vi "菜单-执行.vi"(8 "error in (no error)":errorcluster caption="错误输入（无错误）", 11 "程序响应 输入":refnum<class "程序响应.lvclass">) -> (0 "error out":errorcluster caption="错误输出", 3 "程序响应 输出":refnum<class "程序响应.lvclass">)   [LabVIEW 2020, in "程序响应.lvlib" / "程序响应.lvclass"]
uses:
  D:/SuperPython-master/ScintillaNET.dll
  ScintillaNET.dll
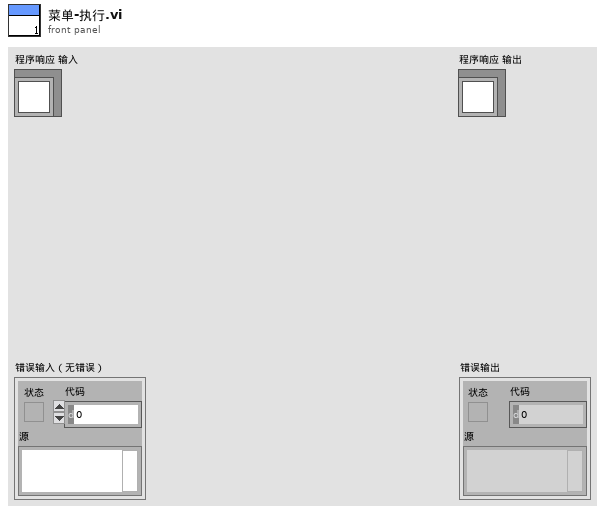
[diagram p1: front panel]
types:
  T1 = enum16{"open", "replace", "create", "open or create", "replace or create", "replace or create with confirmation"}
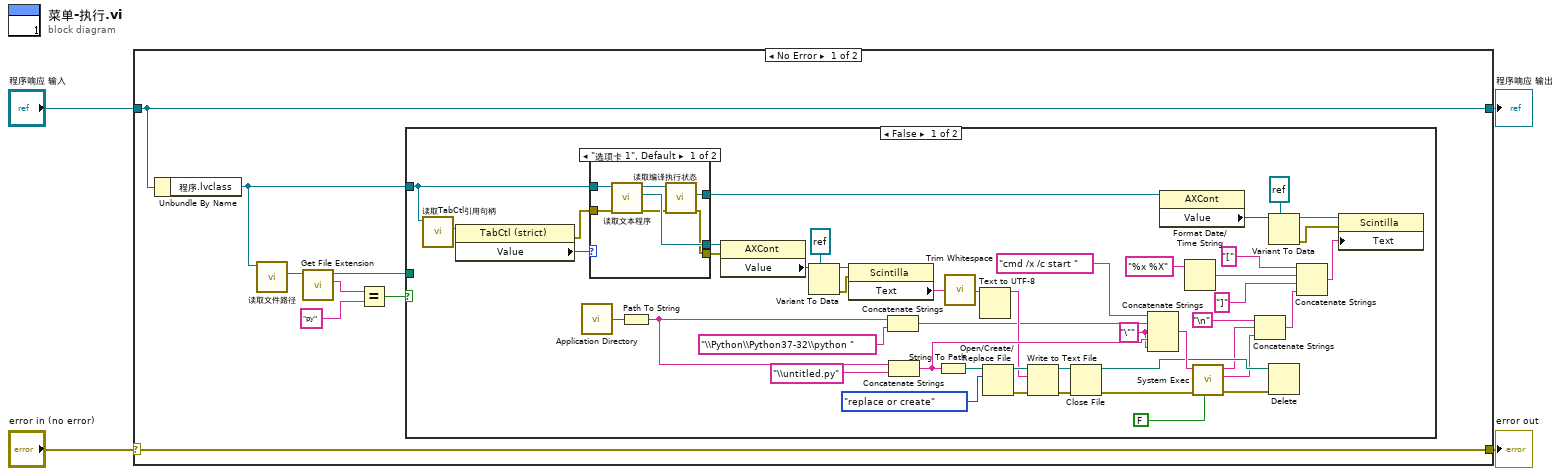
[diagram p0: block diagram]
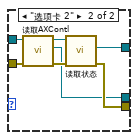
[diagram p2: hidden frame]
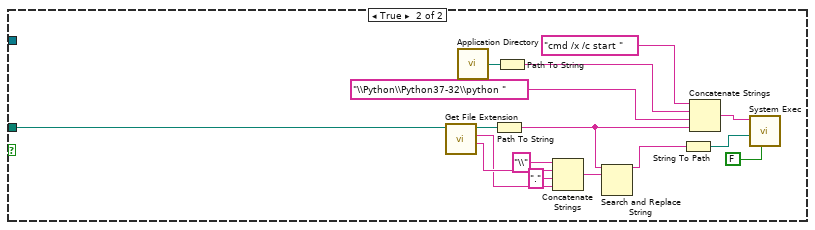
[diagram p3: hidden frame]
diagram:
  n1 = case shown="No Error" "error in (no error)" {
    selector: "error in (no error)" -> [w12 w89]
    tunnel: [w12 w89] -> w3
    tunnel: [w11 w88] -> w1
    tunnel: "程序响应 输入" -> [w11 w88]
    frame No Error {
      n2 = Unbundle By Name(w11) -> ("程序.lvclass"=w10:refnum<class "程序.lvclass">)
      n3 = call-dynamic "读取文件路径.vi"("程序输入"=w10) -> ("文件路径"=w9:path)  [unwired: 8 in, 2 out]
      n4 = call <vilib>:"Get File Extension.vi"("file"=w9) -> ("lowercase file extension"=w8:string, "dup file"=w5:path)  [unwired: 6 in, 3 out]
      n5 = Equal?(x=w8, y="py") -> (x = y?=w6:bool)
      n6 = case shown="False" w6 {
        tunnel: w10 -> [w19 _]
        tunnel: w5 -> [_ w80]
        frame False {
          w17 = "\"" ("字符串")
          n7 = call-dynamic "读取TabCtl引用句柄.vi"("程序输入"=w19) -> ("TabCtl引用句柄"=w23:refnum<vi>)  [unwired: 8 in, 2 out]
          n8 = property class="TabCtl (strict)"(reference=w23) -> (error out=w25:errorcluster, "Value"=w24:enum32{"选项卡 1", "选项卡 2"})  [unwired: 1 in, 1 out]
          n9 = call <vilib>:"Application Directory.vi"() -> ("Application Directory"=w58:path)
          n10 = case shown="\"选项卡 1\", Default" w24 {
            tunnel: [w64 w66] -> w21
            tunnel: [w60 w67] -> w20
            tunnel: [w63 w68] -> w22
            tunnel: w19 -> [w62 w72]
            tunnel: w25 -> [w59 w69]
            frame "选项卡 1", Default {
              n11 = call-dynamic "读取文本程序.vi"("error in (no error)"=w59, "程序输入"=w62) -> ("error out"=w61:errorcluster, "文本程序"=w64:refnum<vi>, "程序输出"=w65:refnum<class "程序.lvclass">)  [unwired: 7 in]
              n12 = call-dynamic "读取编译执行状态.vi"("error in (no error)"=w61, "程序输入"=w65) -> ("error out"=w60:errorcluster, "编译执行状态"=w63:refnum<vi>)  [unwired: 7 in, 1 out]
            }
            frame "选项卡 2" {
              n13 = call-dynamic "读取AXContl.vi"("error in (no error)"=w69, "程序输入"=w72) -> ("error out"=w70:errorcluster, "AXContl"=w66:refnum<vi>, "程序输出"=w71:refnum<class "程序.lvclass">)  [unwired: 7 in]
              n14 = call-dynamic "读取状态.vi"("error in (no error)"=w70, "程序输入"=w71) -> ("error out"=w67:errorcluster, "状态"=w68:refnum<vi>)  [unwired: 7 in, 1 out]
            }
          }
          n15 = Path To String(path=w58) -> (string=w14:string)
          n16 = property class="AXCont"(reference=w21, error in=w20) -> ("Value"=w35:variant)  [unwired: 2 out]
          n17 = Variant To Data(type=refnum<k24> refnum ("文本编辑"), Variant=w35) -> (data=w32:refnum<k24>, error out=w33:errorcluster)  [unwired: 1 in]
          n18 = property class="Scintilla"(reference=w32, error in=w33) -> ("Text"=w31:string)  [unwired: 2 out]
          n19 = Concatenate Strings(w14, "\\Python\\Python37-32\\python " ("字符串")) -> (w15:string)
          n20 = Concatenate Strings(w14, "\\untitled.py" ("字符串")) -> (w49:string)
          n21 = String To Path(string=w49) -> (path=w56:path)
          n22 = call <vilib>:"Trim Whitespace.vi"("string"=w31) -> ("trimmed string"=w37:string)  [unwired: 1 in]
          n23 = Text to UTF-8(11:w37) -> (3:w36:string)  [unwired: 2 in, 1 out]
          n24 = Open/Create/Replace File(file path (use dialog)=w56, operation (0:open)=T1."replace or create" ("操作(0:open)")) -> (refnum out=w55:refnum<file>, error out=w54:errorcluster)  [unwired: 4 in, 1 out]
          n25 = Write to Text File(file (use dialog)=w55, text=w36, error in=w54) -> (refnum out=w53:refnum<file>, error out=w52:errorcluster)  [unwired: 1 in, 1 out]
          n26 = Close File(refnum=w53, error in=w52) -> (path=w46:path, error out=w50:errorcluster)
          n27 = Concatenate Strings("cmd /x /c start " ("字符串"), w15, w17, w49, w17) -> (w48:string)
          n28 = property class="AXCont"(reference=w22) -> ("Value"=w27:variant)  [unwired: 1 in, 2 out]
          n29 = Format Date/Time String(time format string (%c)="%x %X" ("时间格式字符串(%c)")) -> (date/time string=w42:string)  [unwired: 2 in]
          n30 = call <vilib>:"System Exec.vi"("run minimized? (F)"=FALSE, "error in (no error)"=w50, "command line"=w48) -> ("error out"=w47:errorcluster, "standard error"=w45:string, "standard output"=w44:string)  [unwired: 5 in, 1 out]
          n31 = Concatenate Strings("\n", w44, w45) -> (w38:string)
          n32 = Variant To Data(type=refnum<k24> refnum ("文本编辑"), Variant=w27) -> (data=w30:refnum<k24>, error out=w29:errorcluster)  [unwired: 1 in]
          n33 = Delete(path (use dialog)=w46, error in=w47) -> ()  [unwired: 3 in, 3 out]
          n34 = Concatenate Strings("[" ("字符串"), w42, "]" ("字符串"), w38) -> (w26:string)
          n35 = property class="Scintilla"(reference=w30, error in=w29, "Text"=w26) -> ()  [unwired: 2 out]
        }
        frame True {
          n36 = call <vilib>:"Get File Extension.vi"("file"=w80) -> ("filename without extension"=w85:string, "lowercase file extension"=w84:string)  [unwired: 6 in, 3 out]
          n37 = call <vilib>:"Application Directory.vi"() -> ("Application Directory"=w76:path)
          n38 = Path To String(path=w80) -> (string=w82:string)
          n39 = Path To String(path=w76) -> (string=w75:string)
          n40 = Concatenate Strings("\\" ("字符串"), w85, "." ("字符串"), w84) -> (w77:string)
          n41 = Search and Replace String(input string=w82, search string=w77) -> (result string=w78:string)  [unwired: 6 in, 3 out]
          n42 = String To Path(string=w78) -> (path=w79:path)
          n43 = Concatenate Strings("cmd /x /c start " ("字符串"), w75, "\\Python\\Python37-32\\python " ("字符串"), w82) -> (w87:string)
          n44 = call <vilib>:"System Exec.vi"("run minimized? (F)"=FALSE, "working directory"=w79, "command line"=w87) -> ()  [unwired: 5 in, 4 out]
        }
      }
    }
    frame Error {
    }
  }
  "error out" <- w3
  "程序响应 输出" <- w1
